vi "Configure Scale of Magnetic Field Output.vi"(8 "error in (no error)":errorcluster, 10 "Local Horizontal Field Strength ( 0 )":i32 min=0 max=6000, 11 "VISA resource name":refnum<visa-resource-name>) -> (0 "error out":errorcluster, 3 "VISA resource out":refnum<visa-resource-name>)   [LabVIEW 2011, in "Ocean Server OS4000.lvlib"]
doc: "Set the value of the local horizontal field strength of the earth’s magnetic field.\n\nAfter you enter this and do a calibration the compass will output 3 axis magnetic sensor values in milliguass. The local H field strength can be estimated using the NOAA\nworld magnetic model for you local area."
uses:
  Ocean Server OS4000.lvlib
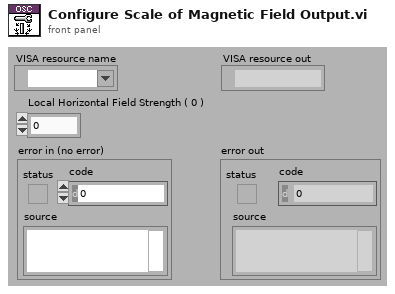
[diagram p1: front panel]
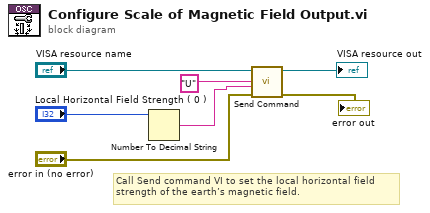
[diagram p0: block diagram]
diagram:
  # "Call Send command VI to set the local horizontal field\nstrength of the earth’s magnetic field."
  n1 = Number To Decimal String(number="Local Horizontal Field Strength ( 0 )") -> (decimal integer string=w1:string)  [unwired: 1 in]
  n2 = call "Send Command.vi"("error in (no error)"="error in (no error)", "Value"=w1, "Message"="U", "VISA resource name"="VISA resource name") -> ("error out"=→"error out":errorcluster, "VISA resource out"=→"VISA resource out":refnum<visa-resource-name>)  [unwired: 6 in]
